vi "Correct_Position_infoY-15_TF.vi"() -> (0 "error out":errorcluster, 4 "Path":path)   [LabVIEW 2012]
panel:
  out "File Changed":bool
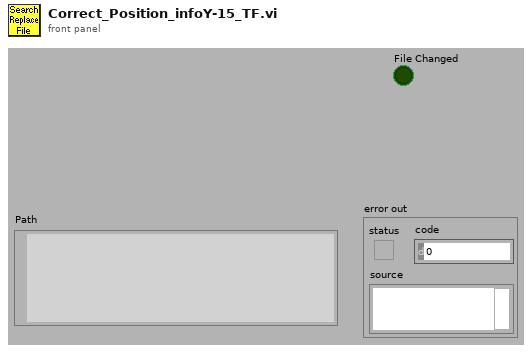
[diagram p1: front panel]
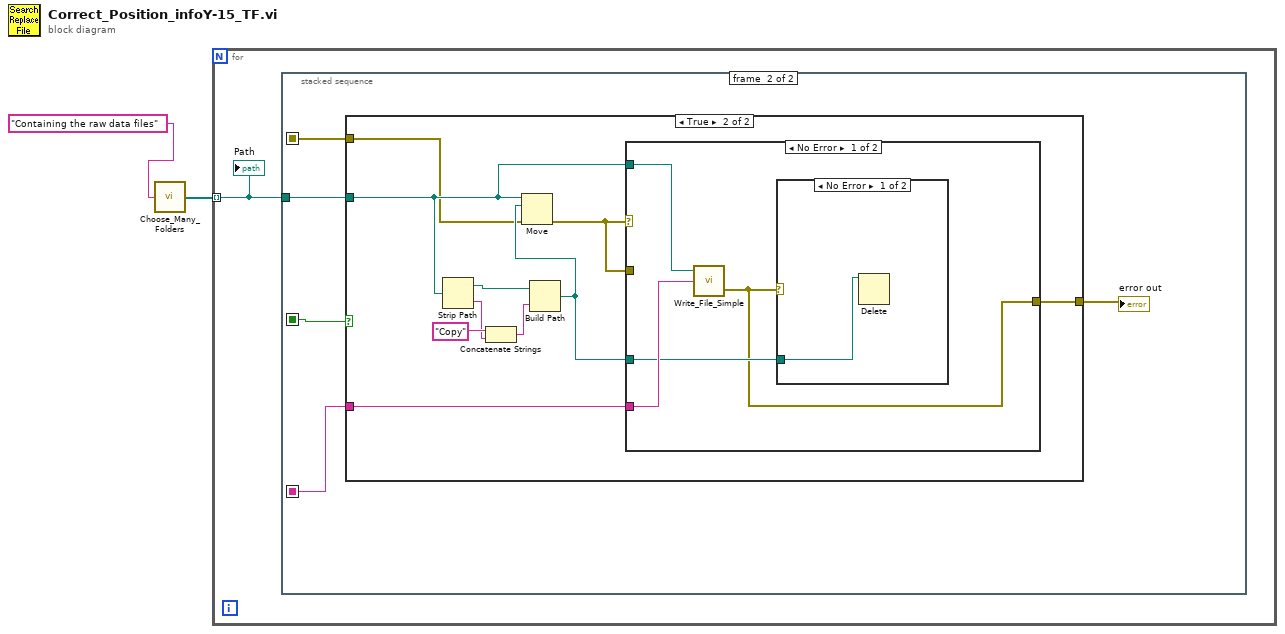
[diagram p0: block diagram]
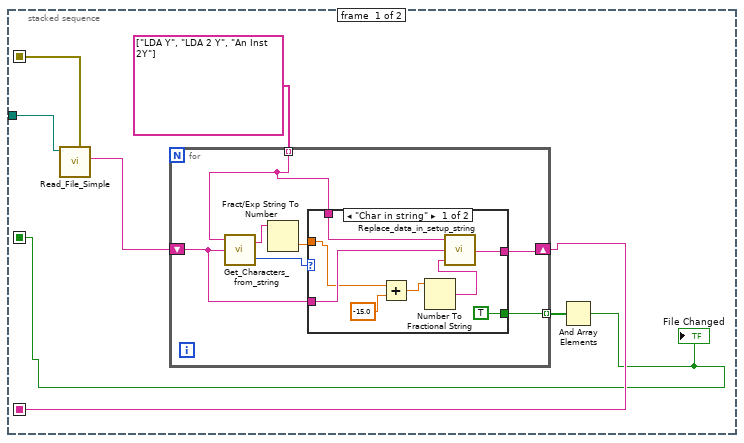
[diagram p2: hidden frame]
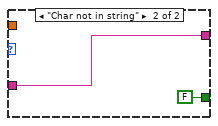
[diagram p3: hidden frame]
diagram:
  n1 = call "Choose_Many_Folders.vi"("Purpose of choosing folder"="Containing the raw data files") -> ("Files"=w1:path[])
  n2 = for {
    tunnel: w1 -> [w3] mode=indexing
    n3 = stacked-sequence {
      seq-local: [w9 _] -> [_ w28]
      seq-local: [w7 _] -> [_ w30]
      seq-local: [w4 _] -> [_ w29]
      tunnel: w3 -> [w10 w32]
      frame #0 {
        n4 = call "Read_File_Simple.vi"("Filename"=w10) -> ("error out"=w9:errorcluster, "string"=w6:string)  [unwired: 4 in, 4 out]
        n5 = for {
          shift-right: [w16] -> w7
          shift-left: w6 -> [w17]
          tunnel: string[] ["LDA Y", "LDA 2 Y", "An Inst 2Y"] -> [w11] mode=indexing
          tunnel: [w14] -> w5 mode=indexing
          n6 = call "Get_Characters_from_string.vi"("Input string"=w17, "Variable name"=w11) -> ("Status"=w15:enum16{"Char in string", "Char not in string"}, "Value"=w13:string)  [unwired: 1 in]
          n7 = Fract/Exp String To Number(string=w13) -> (number=w12:dbl)  [unwired: 3 in, 1 out]
          n8 = case shown="\"Char in string\"" w15 {
            tunnel: w17 -> [w25 w27]
            tunnel: [w18 w27] -> w16
            tunnel: w12 -> [w22 _]
            tunnel: [TRUE FALSE] -> w14
            tunnel: w11 -> [w23 _]
            frame "Char in string" {
              n9 = Add(x=w22, y=-15.0) -> (x+y=w20:dbl)
              n10 = Number To Fractional String(number=w20) -> (F-format string=w19:string)  [unwired: 3 in]
              n11 = call "Replace_data_in_setup_string.vi"("New data string"=w19, "Input string"=w25, "Variable name"=w23) -> ("Appended string"=w18:string)
            }
            frame "Char not in string" {
            }
          }
        }
        n12 = And Array Elements(Boolean array=w5) -> (logical AND=w4:bool)
        "File Changed" <- w4
      }
      frame #1 {
        n13 = case shown="True" w29 {
          tunnel: w32 -> [_ w39]
          tunnel: w30 -> [_ w38]
          tunnel: [w33 w36] -> w31
          tunnel: w28 -> [w33 w34]
          frame False {
          }
          frame True {
            n14 = Strip Path(path=w39) -> (stripped path=w40:path, name=w42:string)
            n15 = Concatenate Strings("Copy" ("name or relative path"), w42) -> (w41:string)
            n16 = Build Path(base path=w40, name or relative path=w41) -> (appended path=w37:path)
            n17 = Move(source path=w39, error in=w34, 10:w37) -> (error out=w35:errorcluster)  [unwired: 2 in, 2 out]
            n18 = case shown="No Error" w35 {
              tunnel: w39 -> [w47 _]
              tunnel: w38 -> [w46 _]
              tunnel: w37 -> [w45 _]
              tunnel: [w44 w49] -> w36
              tunnel: w35 -> [_ w49]
              frame No Error {
                n19 = call "Write_File_Simple.vi"("character string"=w46, "file path"=w47) -> ("error out"=w44:errorcluster)  [unwired: 1 in, 1 out]
                n20 = case shown="No Error" w44 {
                  tunnel: w45 -> [w48 _]
                  frame No Error {
                    n21 = Delete(path (use dialog)=w48) -> ()  [unwired: 4 in, 3 out]
                  }
                  frame Error {
                  }
                }
              }
              frame Error {
              }
            }
          }
        }
        "error out" <- w31
      }
    }
    "Path" <- w3
  }
